vi "ReadAnalogCont.vi"() -> ()   [LabVIEW 2015]
panel:
  out "x-y":u32
  out "millisecond timer value":u32
  out "out":u16
  out "YLDRMErrorOut":errorcluster
  out "YLDRMPortOut":refnum<visa-resource-name>
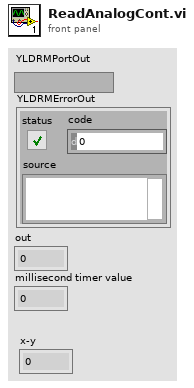
[diagram p1: front panel]
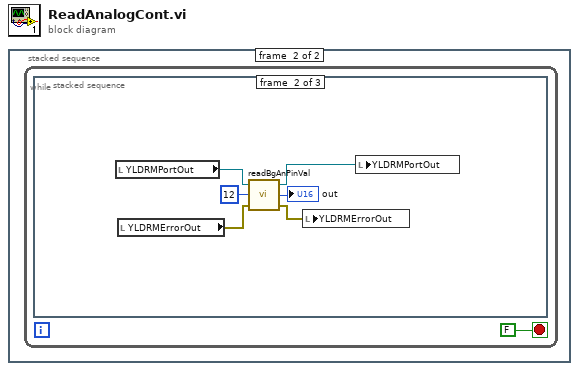
[diagram p0: block diagram]
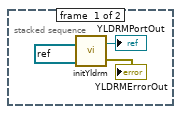
[diagram p2: hidden frame]
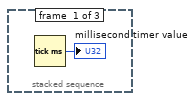
[diagram p3: hidden frame]
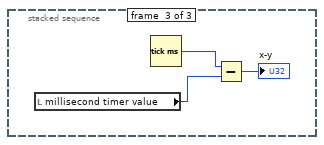
[diagram p4: hidden frame]
diagram:
  n1 = stacked-sequence {
    frame #0 {
      n2 = call "initYldrm.vi"("YLDRMPortInp"=refnum<visa-resource-name> "COM9") -> ("YLDRMPortOut"=→"YLDRMPortOut":refnum<visa-resource-name>, "YLDRMErrorOut"=→"YLDRMErrorOut":errorcluster)
    }
    frame #1 {
      n3 = while {
        stop <- FALSE stop-if-true
        n4 = stacked-sequence {
          frame #0 {
            n5 = Tick Count (ms)() -> (millisecond timer value=→"millisecond timer value":u32)
          }
          frame #1 {
            n6 = local read "YLDRMPortOut"() -> (w10:refnum<visa-resource-name>)
            n7 = local read "YLDRMErrorOut"() -> (w9:errorcluster)
            n8 = call "readBgAnPinVal.vi"("YLDRMErrorInp"=w9, "pin"=u8 12, "YLDRMPortInp"=w10) -> ("YLDRMErrorOut"=w6:errorcluster, "out"=→"out":u16, "YLDRMPortOut"=w7:refnum<visa-resource-name>)
            n9 = local write "YLDRMErrorOut"(w6) -> ()
            n10 = local write "YLDRMPortOut"(w7) -> ()
          }
          frame #2 {
            n11 = local read "millisecond timer value"() -> (w13:u32)
            n12 = Tick Count (ms)() -> (millisecond timer value=w14:u32)
            n13 = Subtract(x=w14, y=w13) -> (x-y=→"x-y":u32)
          }
        }
      }
    }
  }
